vi "HFRR ADV v013 new software.vi"() -> ()   [LabVIEW 2025] (continued)
                              frame #4 {
                                n2582 = local write "Command"("HE;0" ("Command")) -> ()
                              }
                            }
                          }
                        }
                      }
                      frame True {
                      }
                    }
                    n2583 = local write "String 14"("Test will autostart once parameters reach the set value." ("String 14")) -> ()
                  }
                  frame True {
                    (unwired) FALSE ("Visible")
                    n2584 = property on="Stroke 2" class="DigNum (strict)"("Visible"=TRUE) -> ()  [unwired: 2 in, 2 out]
                    n2585 = property on="STOP 2" class="Bool (strict)"("Disabled"=u8 2) -> ()  [unwired: 2 in, 2 out]
                    n2586 = local write "String 14"(" Running....." ("String 14")) -> ()
                    n2587 = property on="Heater Button" class="Bool (strict)"("DisabledEnum"=T17."Disabled and Grayed Out" ("Disabled")) -> ()  [unwired: 2 in, 2 out]
                    n2588 = property on="Humidity" class="Bool (strict)"("DisabledEnum"=T17."Disabled and Grayed Out" ("Disabled")) -> ()  [unwired: 2 in, 2 out]
                    n2589 = case shown="True" "Start Time" {
                      selector: "Start Time" -> [_ w3108]
                      frame False {
                      }
                      frame True {
                        n2590 = Not(x=w3108) -> (.not. x?=w3107:bool)
                        n2591 = local write "Start Time"(w3107) -> ()
                        n2592 = local read "EVENT LOG"() -> (w3109:string)
                        n2593 = call "Event Log.vi"("Content"="Test in progress", "EVENT LOG"=w3109) -> ("EVENT LOG"=w3111:string)  [unwired: 8 in, 1 out]
                        n2594 = local write "EVENT LOG"(w3111) -> ()
                      }
                    }
                    n2595 = disable-structure shown="Enabled" {
                      disable-tunnel: [w3100 w3106] -> w3089
                      frame Disabled {
                        n2596 = local read "Set Hz"() -> (w3103:dbl)
                        n2597 = call <vilib>:"Uniform White Noise Waveform.vi"() -> ("signal out"=w3102:waveform(dbl))  [unwired: 10 in, 1 out]
                        n2598 = Random Number (0-1)() -> (number: 0 to 1=w3099:dbl)
                        n2599 = Add(x=w3103, y=w3102) -> (x+y=w3101:waveform(dbl))
                        n2600 = Multiply(x=ext 0.01 ("y"), y=w3099) -> (x*y=w3097:ext)
                        n2601 = Multiply(x=w3101, y=w3097) -> (x*y=w3100:waveform(ext))
                      }
                      frame Enabled {
                        n2602 = call-poly <vilib>:"Random Number (Range).vi"("lower bound (0)"=49.89, "upper bound (100)"=50.8) -> ("number"=w3106:dbl)  [unwired: 9 in]
                      }
                    }
                    "StartFlg" <- TRUE ("StartFlg")
                  }
                }
                n2603 = case shown="True" w3060 {
                  frame False {
                  }
                  frame True {
                    n2604 = local write "clk"(10.0 ("clk")) -> ()
                    n2605 = Get Date/Time In Seconds() -> (seconds since 1Jan1904=w3114:timestamp)
                    n2606 = To Double Precision Float(number=w3114) -> (double precision float=w3112:dbl)
                    n2607 = local write "acq timer"(w3112) -> ()
                    n2608 = local write "act save time"(w3112) -> ()
                  }
                }
                n2609 = call "Elapsed Time"("Time Target (s)"="Countdown", "Reset"=w3049) -> ("Elapsed Time (s)"=w3054:dbl, "Time has Elapsed"=w3052:bool)  [unwired: 10 in, 6 out]
                "Countdown 2" <- w3054
                n2610 = Subtract(x=w3054, y=2.0) -> (x-y=w3057:dbl)
                n2611 = Less?(x=w3057, y="Countdown") -> (x < y?=w3055:bool)
                n2612 = And(x=w3055, y=w3052) -> (x .and. y?=w3051:bool)
                n2613 = case shown="True" w3051 {
                  frame False {
                  }
                  frame True {
                    (unwired) dbl[] [] ("History Data")
                    n2614 = local write "Engage"(FALSE ("Engage")) -> ()
                    n2615 = local write "RUN"(TRUE ("RUN")) -> ()
                    n2616 = local read "Humidity ( %RH )"() -> (→"Rh Before":dbl)
                  }
                }
                n2617 = local read "Test \nStatus"() -> (w3047:bool)
                n2618 = Select(t=w3045, s=w3047, f=0.0) -> (s? t:f=w3046:dbl)
                n2619 = local write "Frequency ( Hz )"(w3046) -> ()
              }
              frame #1 {
                w3137 = 1000000.0 ("x")
                # "HC;1/0\nST;VALUE"
                # "Elapsed time\ncof\nstroke\nAir temp\nTemp\nHumidity"
                # "acq timer\n\nact save time"
                # "convert to microseconds"
                n2620 = local read "COUNT"() -> (w3120:i32)
                n2621 = local read "Rate"() -> (w3133:dbl)
                n2622 = Divide(x=w3137, y=w3133) -> (x/y=w3138:dbl)
                n2623 = Greater Or Equal?(x=w3120, y=250) -> (x >= y?=w3119:bool)
                n2624 = Get Date/Time In Seconds() -> (seconds since 1Jan1904=w3140:timestamp)
                n2625 = case shown="True" w3119 {
                  frame False {
                    n2626 = local read "COUNT"() -> (w3141:i32)
                    n2627 = Increment(x=w3141) -> (x+1=w3142:i32)
                    n2628 = local write "COUNT"(w3142) -> ()
                  }
                  frame True {
                    n2629 = local write "COUNT"(0 ("COUNT")) -> ()
                  }
                }
                n2630 = local read "Samplingtime 2"() -> (w3118:dbl)
                n2631 = local read "act save time"() -> (w3135:dbl)
                n2632 = Divide(x=w3138, y=w3137) -> (x/y=w3136:dbl)
                n2633 = To Double Precision Float(number=w3140) -> (double precision float=w3129:dbl)
                n2634 = Add(x=w3135, y=w3118) -> (x+y=w3134:dbl)
                n2635 = local read "acq timer"() -> (w3139:dbl)
                n2636 = local read "COUNT"() -> (w3122:i32)
                n2637 = Greater Or Equal?(x=w3129, y=w3134) -> (x >= y?=w3117:bool)
                n2638 = Multiply(x=w3136, y=w3122) -> (x*y=w3128:dbl)
                n2639 = Subtract(x=w3129, y=w3139) -> (x-y=w3131:dbl)
                n2640 = local read "Save"() -> (w3132:bool)
                n2641 = Add(x=w3131, y=w3128) -> (x+y=w3115:dbl)
                "Elapsed time 3" <- w3115
                n2642 = And(x=w3117, y=w3132) -> (x .and. y?=w3130:bool)
                n2643 = Divide(x=w3115, y=60.0) -> (x/y=w3126:dbl)
                n2644 = local read "Test \nStatus"() -> (w3116:bool)
                n2645 = local read "clk"() -> (w3123:dbl)
                n2646 = Equal?(x=w3123, y=10.0) -> (x = y?=w3125:bool)
                n2647 = case shown="True" w3130 {
                  tunnel: w3129 -> [_ w3253]
                  tunnel: [FALSE ("Boolean 2") TRUE ("Boolean 2")] -> _
                  frame False {
                  }
                  frame True {
                    w3207 = ";" ("Substring")
                    # "Pid out/\nFreq response value"
                    n2648 = local write "act save time"(w3253) -> ()
                    n2649 = local read "FILE"() -> (w3201:string)
                    n2650 = call "file check.vi"("file name in"=w3201) -> ("error out"=w3204:errorcluster, "file name out"=w3199:string)  [unwired: 9 in]
                    n2651 = local read "LVDT STROKE"() -> (w3196:dbl)
                    n2652 = local read "Add up Stroke"() -> (w3194:dbl)
                    n2653 = call "FILE PATH CREATION.vi"("error in"=w3204, "FILE NAME :"=w3199) -> ("FILE OUT"=w3202:path)  [unwired: 8 in, 1 out]
                    n2654 = Concatenate Strings(w3199, ".dgf" ("Substring")) -> (w3203:string)
                    n2655 = Subtract(x=w3196, y=w3194) -> (x-y=w3195:dbl)
                    n2656 = Absolute Value(x=w3195) -> (abs(x)=w3193:dbl)
                    n2657 = local read "FF 2"() -> (→"Frictional Force ( N )" →"Frictional Force ( N )":dbl)
                    n2658 = Build Path(base path=w3202, name or relative path=w3203) -> (appended path=w3198:path)
                    n2659 = local read "COF 2"() -> (w3212:dbl)
                    "cof" <- w3212
                    "Coefficient of Friction" <- w3212
                    "COF 4" <- w3212
                    "Coefficient of Friction" <- w3212
                    n2660 = local read "TEMP"() -> (w3215:dbl)
                    "Temp" <- w3215
                    "Temperature ( Deg C )" <- w3215
                    n2661 = local read "Humidity ( %RH )"() -> (w3214:dbl)
                    "Humidity ( %RH )" <- w3214
                    "Humidity ( %RH )" <- w3214
                    n2662 = local read "Frequency ( Hz )"() -> (w3221:dbl)
                    n2663 = call <vilib>:"Mean PtByPt.vi"("x"=w3193, "sample length"=10) -> ("mean"=w3192:dbl)  [unwired: 2 in, 1 out]
                    n2664 = local read "Elapsed time"() -> (w3246:dbl)
                    n2665 = local read "AIR TEMP"() -> (w3219:dbl)
                    n2666 = local read "PID-out"() -> (w3224:dbl)
                    n2667 = local write "Temperature ( Deg C )"(w3215) -> ()
                    n2668 = Number To Fractional String(number=w3192, width (-)=i16 9 ("precision (6)"), precision (6)=i16 6) -> (F-format string=w3239:string)  [unwired: 1 in]
                    n2669 = Number To Fractional String(number=w3219, width (-)=i16 9 ("precision (6)"), precision (6)=i16 3) -> (F-format string=w3238:string)  [unwired: 1 in]
                    n2670 = Number To Fractional String(number=w3215, width (-)=i16 9 ("precision (6)"), precision (6)=i16 3) -> (F-format string=w3235:string)  [unwired: 1 in]
                    n2671 = Number To Fractional String(number=w3214, width (-)=i16 9 ("precision (6)"), precision (6)=i16 3) -> (F-format string=w3232:string)  [unwired: 1 in]
                    n2672 = Number To Fractional String(number=0.0, width (-)=i16 9 ("precision (6)"), precision (6)=i16 3) -> (F-format string=w3229:string)  [unwired: 1 in]
                    n2673 = Number To Fractional String(number=w3224, width (-)=i16 9 ("precision (6)"), precision (6)=i16 3) -> (F-format string=w3225:string)  [unwired: 1 in]
                    n2674 = Number To Fractional String(number=w3221, width (-)=i16 9 ("precision (6)"), precision (6)=i16 3) -> (F-format string=w3220:string)  [unwired: 1 in]
                    n2675 = Number To Fractional String(number=w3212, width (-)=i16 9 ("precision (6)"), precision (6)=i16 6) -> (F-format string=w3247:string)  [unwired: 1 in]
                    n2676 = Number To Fractional String(number=w3246, width (-)=i16 14 ("precision (6)"), precision (6)=i16 3) -> (F-format string=w3248:string)  [unwired: 1 in]
                    n2677 = Bundle("y"=1.02, "mean"=w3192, "y"=0.98) -> (w3213:cluster{"y":dbl, "mean":dbl, "y":dbl})  [unwired: 1 in]
                    n2678 = Number To Fractional String(number="Ambient Humidity :", width (-)=i16 9 ("precision (6)"), precision (6)=i16 6) -> (F-format string=w3205:string)  [unwired: 1 in]
                    n2679 = local read "RUN"() -> (w3211:bool)
                    n2680 = case shown="True" w3211 {
                      tunnel: w3213 -> [_ w3258]
                      tunnel: w3192 -> [_ w3257]
                      tunnel: w3192 -> [_ w3255]
                      tunnel: w3192 -> [_ w3256]
                      frame False {
                      }
                      frame True {
                        "Stroke ( mm )" <- w3258
                        "Stroke ( mm )" <- w3258
                        "Stroke 4" <- w3257
                        "Stroke 3" <- w3255
                        "Stroke 2" <- w3256
                        "measured_stroke" <- w3255
                      }
                    }
                    n2681 = Concatenate Strings(w3248, w3207, w3247, w3207, w3239, w3207, w3238, w3207, w3235, w3207, w3232, w3207, w3229, w3207, w3225, w3207, w3220, w3207, w3205, "\r") -> (w3245:string)
                    n2682 = call <vilib>:"Write Characters To File.vi"("append to file? (new file:F)"=TRUE, "character string"=w3245, "file path (dialog if empty)"=w3198) -> ()  [unwired: 2 in, 1 out]
                    "refresh flag" <- TRUE ("refresh flag")
                  }
                }
                n2683 = case shown="True" w3116 {
                  tunnel: w3126 -> [_ w3152]
                  tunnel: w3131 -> [_ w3162]
                  tunnel: [0.0 w3158] -> _
                  tunnel: w3125 -> [_ w3157]
                  tunnel: [0.0 w3156] -> _
                  tunnel: w3115 -> [_ w3156]
                  tunnel: w3129 -> [w3145 _]
                  frame False {
                    n2684 = local write "acq timer"(w3145) -> ()
                    n2685 = local write "Test Duration Status"(0.0 ("Test Duration Status")) -> ()
                  }
                  frame True {
                    n2686 = local read "Set Hz"() -> (w3159:dbl)
                    n2687 = local write "Elapsed time"(w3152) -> ()
                    n2688 = local read "test time"() -> (w3151:dbl)
                    n2689 = Multiply(x=w3162, y=w3159) -> (x*y=w3161:dbl)
                    n2690 = case shown="False" w3157 {
                      tunnel: w3161 -> [w3163 _]
                      tunnel: [w3163 1.0] -> w3158
                      frame False {
                        n2691 = local write "Cycles elapsed"(w3163) -> ()
                      }
                      frame True {
                      }
                    }
                    n2692 = Greater?(x=w3152, y=w3151) -> (0:w3160:bool)
                    n2693 = Subtract(x=w3151, y=w3152) -> (x-y=w3150:dbl)
                    "time" <- w3150
                    n2694 = Multiply(x=w3150, y=60.0) -> (x*y=w3149:dbl)
                    n2695 = local write "Time Remaining"(w3149) -> ()
                    n2696 = local write "Remaining Time"(w3149) -> ()
                    n2697 = case shown="True" w3160 {
                      frame False {
                      }
                      frame True {
                        n2698 = stacked-sequence {
                          frame #0 {
                            w3168 = T17."Enabled" ("Disabled")
                            w3167 = FALSE ("TEST FILE NAM,E SAVED")
                            w3169 = "" ("FILE")
                            w3170 = TRUE ("Visible")
                            n2699 = local write "Humidity"(FALSE ("Humidity")) -> ()
                            n2700 = local write "RUN"(FALSE ("OK Button 2")) -> ()
                            n2701 = local write "Heater Button"(FALSE ("Heater Button")) -> ()
                            n2702 = local write "Auto Start Test"(FALSE ("Auto Start Test")) -> ()
                            n2703 = local write "TestCompFlg"(TRUE ("StpFlg")) -> ()
                            n2704 = local read "Humidity ( %RH )"() -> (→"Rh After":dbl)
                            n2705 = property on="STOP 2" class="Bool (strict)"("Disabled"=u8 0) -> ()  [unwired: 2 in, 2 out]
                            n2706 = local read "EVENT LOG"() -> (w3175:string)
                            n2707 = call "Event Log.vi"("Content"="Test Completed", "EVENT LOG"=w3175) -> ("EVENT LOG"=w3174:string)  [unwired: 8 in, 1 out]
                            n2708 = property on="RUN" class="Bool (strict)"("Visible"=w3170) -> ()  [unwired: 2 in, 2 out]
                            n2709 = property on="Auto Start Test" class="Bool (strict)"("Visible"=w3170) -> ()  [unwired: 2 in, 2 out]
                            n2710 = local write "Batch Ref Num :"(w3169) -> ()
                            n2711 = local write "FILE"(w3169) -> ()
                            n2712 = local write "EVENT LOG"(w3174) -> ()
                            n2713 = local write "TEST FILE NAM,E SAVED"(w3167) -> ()
                            n2714 = local write "Fuel Discription :"(w3169) -> ()
                            n2715 = local write "START TEMP"(w3167) -> ()
                            n2716 = local write "Remarks :"(w3169) -> ()
                            n2717 = local write "Main Dashboard Buttons"(T1."Imaging" ("Main Dashboard Buttons")) -> ()
                            n2718 = local write "Main Tab"(T2."Adv Scar" ("Main Tab")) -> ()
                            n2719 = property on="FRICVALZ 2" class="Bool (strict)"("DisabledEnum"=w3168) -> ()  [unwired: 2 in, 2 out]
                            n2720 = property on="FRICVALZ 3" class="Bool (strict)"("DisabledEnum"=w3168) -> ()  [unwired: 2 in, 2 out]
                            n2721 = property on="FRICVALZ 4" class="Bool (strict)"("DisabledEnum"=w3168) -> ()  [unwired: 2 in, 2 out]
                          }
                          frame #1 {
                            n2722 = Wait (ms)(milliseconds to wait=u32 1500) -> ()  [unwired: 1 out]
                          }
                          frame #2 {
                            n2723 = local write "Command"("VC;0") -> ()
                          }
                          frame #3 {
                            n2724 = Wait (ms)(milliseconds to wait=u32 1500) -> ()  [unwired: 1 out]
                          }
                          frame #4 {
                            n2725 = local write "Command"("VC;0") -> ()
                          }
                          frame #5 {
                            n2726 = Wait (ms)(milliseconds to wait=u32 1500) -> ()  [unwired: 1 out]
                          }
                          frame #6 {
                            n2727 = local write "Command"("ST;0") -> ()
                          }
                          frame #7 {
                            n2728 = local write "measured_stroke"(0.0 ("measured_stroke")) -> ()
                            n2729 = Wait (ms)(milliseconds to wait=u32 1500) -> ()  [unwired: 1 out]
                          }
                          frame #8 {
                            n2730 = local write "Command"("HE;0") -> ()
                          }
                        }
                      }
                    }
                    n2731 = Divide(x=w3152, y=w3151) -> (x/y=w3155:dbl)
                    n2732 = Multiply(x=w3155, y=100.0) -> (x*y=w3153:dbl)
                    n2733 = local write "Test Duration Status"(w3153) -> ()
                  }
                }
              }
              frame #2 {
                n2734 = case shown="True" "Heater Button" {
                  tunnel: [0.0 ("output") w3281] -> w3259
                  frame False {
                    w3262 = TRUE ("tmpchk")
                    n2735 = local read "TEMP"() -> (w3263:dbl)
                    n2736 = local write "Temp ini"(w3263) -> ()
                    n2737 = local write "Reset 4"(w3262) -> ()
                    n2738 = local write "tmpchk"(w3262) -> ()
                    n2739 = local write "reinit"(TRUE ("reinit")) -> ()
                    n2740 = local write "manual temp log"(TRUE ("manual temp log")) -> ()
                  }
                  frame True {
                    # "Logic to turn off\nthe heater when \ntemp is not rising.\nTime - 60 sec\nDelta t- 5°c"
                    n2741 = local read "Temp ini"() -> (w3270:dbl)
                    n2742 = local read "Auto Start Test"() -> (w3266:bool)
                    n2743 = Less?(x=w3270, y=53.0) -> (x < y?=w3268:bool)
                    n2744 = case shown="False" w3266 {
                      frame False {
                        n2745 = local read "Set Temp"() -> (w3290:dbl)
                        n2746 = local read "TEMP"() -> (w3289:dbl)
                        n2747 = Subtract(x=w3290, y=w3289) -> (x-y=w3288:dbl)
                        n2748 = Absolute Value(x=w3288) -> (abs(x)=w3287:dbl)
                        n2749 = Less?(x=w3287, y=0.5) -> (x < y?=w3285:bool)
                        n2750 = case shown="True" w3285 {
                          tunnel: "manual temp log" -> [_ w3291]
                          frame False {
                          }
                          frame True {
                            n2751 = case shown="True" w3291 {
                              selector: w3291 -> [_ w3292]
                              frame False {
                              }
                              frame True {
                                # "#Event log"
                                n2752 = Not(x=w3292) -> (.not. x?=w3293:bool)
                                n2753 = local write "manual temp log"(w3293) -> ()
                                n2754 = local read "EVENT LOG"() -> (w3296:string)
                                n2755 = call "Event Log.vi"("Content"="Target Temperature reached", "EVENT LOG"=w3296) -> ("EVENT LOG"=w3295:string)  [unwired: 8 in, 1 out]
                                n2756 = local write "EVENT LOG"(w3295) -> ()
                              }
                            }
                          }
                        }
                      }
                      frame True {
                        n2757 = local write "manual temp log"(TRUE ("manual temp log")) -> ()
                      }
                    }
                    n2758 = And(x="tmpchk", y=w3268) -> (x .and. y?=w3271:bool)
                    n2759 = case shown="True" w3271 {
                      frame False {
                      }
                      frame True {
                        n2760 = call "Elapsed Time8"("Time Target (s)"=300.0, "Reset"="Reset 4") -> ("Time has Elapsed"=w3298:bool)  [unwired: 10 in, 7 out]
                        n2761 = flat-sequence {
                          tunnel: w3298 -> [_]
                          frame #0 {
                            n2762 = local write "Reset 4"(FALSE ("Reset 4")) -> ()
                          }
                        }
                        n2763 = case shown="True" w3298 {
                          frame False {
                          }
                          frame True {
                            n2764 = local read "Temp ini"() -> (w3305:dbl)
                            n2765 = Add(x=w3305, y=5.0) -> (x+y=w3303:dbl)
                            n2766 = local read "TEMP"() -> (w3306:dbl)
                            n2767 = Greater?(x=w3306, y=w3303) -> (0:w3304:bool)
                            n2768 = case shown="False" w3304 {
                              frame False {
                                n2769 = local write "Heater Button"(FALSE ("Heater Button")) -> ()
                              }
                              frame True {
                                n2770 = local write "tmpchk"(FALSE ("tmpchk")) -> ()
                              }
                            }
                          }
                        }
                      }
                    }
                    n2771 = local read "Set Temp"() -> (w3279:dbl)
                    n2772 = local read "TEMP"() -> (w3273:dbl)
                    n2773 = call-poly <vilib>:"PID.vi"("reinitialize? (F)"="reinit", "dt (s)"=-1.0, "process variable"=w3273, "setpoint"=w3279) -> ("output"=w3276:dbl)  [unwired: 6 in, 1 out]
                    n2774 = Subtract(x=w3279, y=w3273) -> (x-y=w3280:dbl)
                    n2775 = Add(x=w3279, y=0.5) -> (x+y=w3277:dbl)
                    n2776 = Greater Or Equal?(x=w3273, y=w3277) -> ()  [unwired: 1 out]
                    n2777 = Select(t=0.0, s=FALSE, f=w3276) -> (s? t:f=w3275:dbl)
                    "PID output" <- w3275
                    n2778 = flat-sequence {
                      tunnel: w3275 -> [w3309]
                      tunnel: [w3309] -> w3281
                      frame #0 {
                        n2779 = local write "reinit"(FALSE ("reinit")) -> ()
                      }
                    }
                    n2780 = Bundle(w3280, "output"=w3275, "TEMP"=w3273) -> ()  [unwired: 1 in, 1 out]
                  }
                }
                "PID-out" <- w3259
              }
              frame #3 {
                n2781 = local read "TEMP"() -> (w3311:dbl)
                n2782 = Greater Or Equal?(x=w3311, y="Set Temp 2") -> (x >= y?=w3316:bool)
                n2783 = case shown="True" w3316 {
                  tunnel: [FALSE TRUE] -> w3314
                  frame False {
                  }
                  frame True {
                  }
                }
                "Status 13" <- w3314
                n2784 = And(x=w3314, y="trip1 8") -> (x .and. y?=w3313:bool)
                n2785 = case shown="True" w3313 {
                  frame False {
                    n2786 = local write "Heater Trip Temp"(TRUE ("Heater Trip Temp")) -> ()
                  }
                  frame True {
                    w3319 = FALSE ("OK Button 2")
                    n2787 = case shown="True" "Heater Trip Temp" {
                      selector: "Heater Trip Temp" -> [_ w3321]
                      frame False {
                      }
                      frame True {
                        n2788 = Not(x=w3321) -> (.not. x?=w3320:bool)
                        n2789 = local read "EVENT LOG"() -> (w3324:string)
                        n2790 = local write "Heater Trip Temp"(w3320) -> ()
                        n2791 = call "Event Log.vi"("Content"="Heater Trip", "EVENT LOG"=w3324) -> ("EVENT LOG"=w3323:string)  [unwired: 8 in, 1 out]
                        n2792 = local write "EVENT LOG"(w3323) -> ()
                      }
                    }
                    n2793 = local write "RUN"(w3319) -> ()
                    n2794 = property on="Auto Start Test" class="Bool (strict)"("Value"=w3319) -> ()  [unwired: 2 in, 2 out]
                    n2795 = local write "Heater Button"(w3319) -> ()
                  }
                }
              }
            }
            n2796 = case shown="False" w3040 {
              frame False {
                n2797 = disable-structure shown="Disabled" {
                  frame Disabled {
                    n2798 = stacked-sequence {
                      frame #0 {
                        n2799 = local write "RUN"(FALSE ("OK Button 2")) -> ()
                      }
                      frame #1 {
                      }
                    }
                  }
                  frame Enabled {
                  }
                }
              }
              frame True {
              }
            }
          }
        }
        n2800 = local read "airtempflg"() -> (w2832:bool)
        n2801 = Or(x=w2832, y=w2830) -> (x .or. y?=w2833:bool)
        n2802 = Insert Into Array(array=string[] ["Air Temperature has reached set value,", "Humidity has reached set value,", "Sample Temperaturehas reached set value,", ""], index=0, new element="") -> (w2818:string[])
        n2803 = Build Array(w2823, w2822, w2821) -> (w2819:i32[])
        n2804 = disable-structure shown="Disabled" {
          disable-tunnel: w2833 -> [w2910 _]
          disable-tunnel: w2828 -> [w2909 _]
          disable-tunnel: w2826 -> [w2908 _]
          frame Disabled {
            n2805 = Compound Arithmetic op=AND(w2910, w2909, w2908) -> ()  [unwired: 1 out]
            n2806 = case shown="True" {
              selector: _ -> [_ _]
              frame False {
              }
              frame True {
                w2911 = FALSE ("autostrtflg")
                n2807 = local write "RUN"(TRUE ("RUN")) -> ()
                n2808 = local write "autostrtflg"(w2911) -> ()
                n2809 = local write "autostart"(w2911) -> ()
                n2810 = local write "String 14"(" Running....." ("String 14")) -> ()
              }
            }
          }
          frame Enabled {
          }
        }
        n2811 = for {
          tunnel: w2819 -> [w2961] mode=indexing
          tunnel: w2818 -> [w2960]
          shift-right: [w2957] -> w2817
          shift-left: "" -> [w2959]
          n2812 = Index Array(array=w2960, index=w2961) -> (element=w2958:string)
          n2813 = Concatenate Strings(w2958, w2959) -> (w2957:string)
        }
        n2814 = local write "autostart 2"(w2817) -> ()
        n2815 = local read "Reset Graph"() -> (w2806:bool)
        n2816 = case shown="True" w2806 {
          selector: w2806 -> [_ w2860]
          frame False {
          }
          frame True {
            w2874 = 0.0 ("X Scale.Range:Maximum")
            n2817 = Not(x=w2860) -> (.not. x?=w2859:bool)
            n2818 = local write "Reset Graph"(w2859) -> ()
            n2819 = property on="Electrical Contact Resistance ( % )" class="WFChart (strict)"("XScale.Maximum"=600.0 ("X Scale.Range:Maximum"), "XScale.Minimum"=0.0 ("X Scale.Range:Minimum"), "YScale.Maximum"=100.0 ("Y Scale.Range:Maximum"), "YScale.Minimum"=0.0 ("Y Scale.Range:Minimum")) -> ()  [unwired: 2 in, 2 out]
            n2820 = property on="Frictional Force ( N )" class="WFChart (strict)"("XScale.Maximum"=600.0 ("X Scale.Range:Maximum"), "XScale.Minimum"=0.0 ("X Scale.Range:Minimum"), "YScale.Maximum"=100.0 ("Y Scale.Range:Maximum"), "YScale.Minimum"=0.0 ("Y Scale.Range:Minimum")) -> ()  [unwired: 2 in, 2 out]
            n2821 = property on="Temperature ( Deg C )" class="WFChart (strict)"("XScale.Maximum"=600.0 ("X Scale.Range:Maximum"), "XScale.Minimum"=0.0 ("X Scale.Range:Minimum"), "YScale.Maximum"=100.0 ("Y Scale.Range:Maximum"), "YScale.Minimum"=0.0 ("Y Scale.Range:Minimum")) -> ()  [unwired: 2 in, 2 out]
            n2822 = property on="Humidity ( %RH )" class="WFChart (strict)"("XScale.Maximum"=600.0 ("X Scale.Range:Maximum"), "XScale.Minimum"=0.0 ("X Scale.Range:Minimum"), "YScale.Maximum"=100.0 ("Y Scale.Range:Maximum"), "YScale.Minimum"=0.0 ("Y Scale.Range:Minimum")) -> ()  [unwired: 2 in, 2 out]
            n2823 = property on="Stroke ( mm )" class="WFChart (strict)"("XScale.Maximum"=600.0 ("X Scale.Range:Maximum"), "XScale.Minimum"=0.0 ("X Scale.Range:Minimum"), "YScale.Maximum"=100.0 ("Y Scale.Range:Maximum"), "YScale.Minimum"=0.0 ("Y Scale.Range:Minimum")) -> ()  [unwired: 2 in, 2 out]
            n2824 = property on="Coefficient of Friction" class="WFChart (strict)"("XScale.Maximum"=600.0 ("X Scale.Range:Maximum"), "XScale.Minimum"=0.0 ("X Scale.Range:Minimum"), "YScale.Maximum"=100.0 ("Y Scale.Range:Maximum"), "YScale.Minimum"=0.0 ("Y Scale.Range:Minimum")) -> ()  [unwired: 2 in, 2 out]
            n2825 = property on="Electrical Contact Resistance ( % )" class="WFChart (strict)"("XScale.Minimum"=0.0 ("X Scale.Range:Minimum"), "XScale.Maximum"=600.0 ("X Scale.Range:Maximum"), "YScale.Minimum"=0.0 ("Y Scale.Range:Minimum"), "YScale.Maximum"=100.0 ("Y Scale.Range:Maximum")) -> ()  [unwired: 2 in, 2 out]
            n2826 = property on="Temperature ( Deg C )" class="WFChart (strict)"("XScale.Minimum"=0.0 ("X Scale.Range:Minimum"), "XScale.Maximum"=600.0 ("X Scale.Range:Maximum"), "YScale.Minimum"=0.0 ("Y Scale.Range:Minimum"), "YScale.Maximum"=100.0 ("Y Scale.Range:Maximum")) -> ()  [unwired: 2 in, 2 out]
            n2827 = property on="Coefficient of Friction" class="WFChart (strict)"("XScale.Minimum"=0.0 ("X Scale.Range:Minimum"), "XScale.Maximum"=600.0 ("X Scale.Range:Maximum"), "YScale.Maximum"=1.0 ("X Scale.Range:Minimum"), "YScale.Minimum"=0.0 ("X Scale.Range:Minimum")) -> ()  [unwired: 2 in, 2 out]
            n2828 = property on="Frictional Force ( N )" class="WFChart (strict)"("XScale.Maximum"=600.0 ("X Scale.Range:Maximum"), "XScale.Minimum"=w2874, "YScale.Maximum"=10.0 ("Y Scale.Range:Maximum"), "YScale.Minimum"=w2874) -> ()  [unwired: 2 in, 2 out]
            n2829 = property on="Stroke ( mm )" class="WFChart (strict)"("XScale.Maximum"=600.0 ("X Scale.Range:Maximum"), "XScale.Minimum"=0.0 ("X Scale.Range:Minimum"), "YScale.Maximum"=100.0 ("Y Scale.Range:Maximum"), "YScale.Minimum"=0.0 ("Y Scale.Range:Minimum")) -> ()  [unwired: 2 in, 2 out]
            n2830 = property on="Humidity ( %RH )" class="WFChart (strict)"("XScale.Maximum"=600.0 ("X Scale.Range:Maximum"), "XScale.Minimum"=0.0 ("X Scale.Range:Minimum"), "YScale.Maximum"=100.0 ("Y Scale.Range:Maximum"), "YScale.Minimum"=0.0 ("Y Scale.Range:Minimum")) -> ()  [unwired: 2 in, 2 out]
          }
        }
      }
      frame "Compare Files" {
        # "Elapsed time\ncof\nstroke\nAir temp\nTemp\nHumidity"
        n2831 = case shown="True" "RSTV1 2" {
          frame False {
          }
          frame True {
            n2832 = property on="Humidity ( %RH )" class="XYGraph (strict)"("Y Scale.Display Format:Precision"=u8 0 ("Y Scale.Format & Precision:Precision")) -> ()  [unwired: 2 in, 2 out]
            n2833 = property on="Humidity ( %RH )" class="XYGraph (strict)"("X Scale.Range:Minimum"=0.0, "X Scale.Range:Maximum"=75.0, "Y Scale.Range:Minimum"=48.0, "Y Scale.Range:Maximum"=58.0) -> ()  [unwired: 2 in, 2 out]
          }
        }
        n2834 = case shown="True" "RST CP 2" {
          frame False {
          }
          frame True {
            n2835 = property on="XY Graph 13" class="XYGraph (strict)"("Y Scale.Display Format:Precision"=u8 0 ("Y Scale.Format & Precision:Precision")) -> ()  [unwired: 2 in, 2 out]
            n2836 = property on="XY Graph 13" class="XYGraph (strict)"("X Scale.Range:Minimum"=0.0, "X Scale.Range:Maximum"=75.0, "Y Scale.Range:Minimum"=0.0, "Y Scale.Range:Maximum"=100.0) -> ()  [unwired: 2 in, 2 out]
          }
        }
        n2837 = case shown="True" "RST CP" {
          frame False {
          }
          frame True {
            n2838 = property on="Sample Temperature ( °C )" class="XYGraph (strict)"("Y Scale.Display Format:Precision"=u8 2 ("Y Scale.Format & Precision:Precision")) -> ()  [unwired: 2 in, 2 out]
            n2839 = property on="Sample Temperature ( °C )" class="XYGraph (strict)"("X Scale.Range:Minimum"=0.0, "X Scale.Range:Maximum"=75.0, "Y Scale.Range:Minimum"=58.0, "Y Scale.Range:Maximum"=62.0) -> ()  [unwired: 2 in, 2 out]
          }
        }
        n2840 = case shown="True" "RSTV1 3" {
          frame False {
          }
          frame True {
            n2841 = property on="Air Temperature  ( °C )" class="XYGraph (strict)"("Y Scale.Display Format:Precision"=u8 2 ("Y Scale.Format & Precision:Precision")) -> ()  [unwired: 2 in, 2 out]
            n2842 = property on="Air Temperature  ( °C )" class="XYGraph (strict)"("X Scale.Range:Minimum"=0.0 ("Y Scale.Range:Minimum"), "X Scale.Range:Maximum"=75.0 ("Y Scale.Range:Maximum"), "Y Scale.Range:Minimum"=20.0 ("X Scale.Range:Minimum"), "Y Scale.Range:Maximum"=26.0 ("X Scale.Range:Maximum")) -> ()  [unwired: 2 in, 2 out]
          }
        }
        n2843 = case shown="True" "RSTV1 4" {
          frame False {
          }
          frame True {
            n2844 = property on="Stroke ( mm )" class="XYGraph (strict)"("Y Scale.Display Format:Precision"=u8 2 ("Y Scale.Format & Precision:Precision")) -> ()  [unwired: 2 in, 2 out]
            n2845 = property on="Stroke ( mm )" class="XYGraph (strict)"("X Scale.Range:Minimum"=0.0 ("Y Scale.Range:Maximum"), "X Scale.Range:Maximum"=75.0 ("X Scale.Range:Minimum"), "Y Scale.Range:Minimum"=0.98, "Y Scale.Range:Maximum"=1.02) -> ()  [unwired: 2 in, 2 out]
          }
        }
        n2846 = case shown="True" "rstv2" {
          frame False {
          }
          frame True {
            n2847 = property on="Coefficient Of Friction" class="XYGraph (strict)"("Y Scale.Display Format:Precision"=u8 3 ("Y Scale.Format & Precision:Precision")) -> ()  [unwired: 2 in, 2 out]
            n2848 = property on="Coefficient Of Friction" class="XYGraph (strict)"("X Scale.Range:Minimum"=0.0 ("Y Scale.Range:Maximum"), "X Scale.Range:Maximum"=75.0, "Y Scale.Range:Minimum"=0.0, "Y Scale.Range:Maximum"=1.0 ("X Scale.Range:Minimum")) -> ()  [unwired: 2 in, 2 out]
          }
        }
        n2849 = case shown="True" "RST CP 3" {
          frame False {
          }
          frame True {
            n2850 = property on="Air Temp ( °C ) vs Humidity ( % RH )" class="XYGraph (strict)"("X Scale.Range:Minimum"=18.0, "X Scale.Range:Maximum"=28.0 ("X Scale.Range:Minimum"), "Y Scale.Range:Minimum"=30.0 ("X Scale.Range:Minimum"), "Y Scale.Range:Maximum"=70.0 ("X Scale.Range:Minimum")) -> ()  [unwired: 2 in, 2 out]
          }
        }
        n2851 = case shown="True" "OPEN 1" {
          frame False {
          }
          frame True {
            (unwired) 0  # existing file
            w3600 = "Choose a datalog file to open"  # prompt
            n2852 = local write "OPEN 1"(FALSE ("OPEN 1")) -> ()
            n2853 = String To Path(string="C:\\LAB-IQ\\Data\\") -> (path=w3585:path)
            n2854 = File Dialog(6:"*.dgf" ("pattern"), 7:w3600, 11:w3585) -> (0:w3583:errorcluster, 3:w3591:path)  [unwired: 4 in, 2 out]
            n2855 = Unbundle(w3583) -> ()  [unwired: 3 out]
            n2856 = Strip Path(path=w3591) -> (name=w3590:string)  [unwired: 1 out]
            n2857 = Path To String(path=w3591) -> (string=w3586:string)
            "string1" <- w3586
            n2858 = Match Pattern(string=w3590, regular expression=".dgf") -> (before substring=→"String Control":string)  [unwired: 1 in, 3 out]
            n2859 = Match Pattern(string=w3586, regular expression=".dgf" ("substring (\"\")")) -> (before substring=w3596:string)  [unwired: 1 in, 3 out]
            n2860 = Concatenate Strings(w3596, ".duf" ("Substring")) -> (w3592:string)
            n2861 = String To Path(string=w3592) -> (path=w3597:path)
            n2862 = call <vilib>:"Read Characters From File.vi"("file path (dialog if empty)"=w3597, "start of read offset (chars.:0)"=60 ("start of read offset (chars.: 0)")) -> ("character string"=→"String Control 2":string)  [unwired: 4 in, 3 out]
          }
        }
        n2863 = case shown="True" "OPEN 2" {
          frame False {
          }
          frame True {
            (unwired) 0  # existing file
            w3618 = "Choose a datalog file to open"  # prompt
            n2864 = local write "OPEN 2"(FALSE ("OPEN 1")) -> ()
            n2865 = String To Path(string="C:\\LAB-IQ\\Data\\") -> (path=w3603:path)
            n2866 = File Dialog(6:"*.dgf" ("pattern"), 7:w3618, 11:w3603) -> (0:w3601:errorcluster, 3:w3609:path)  [unwired: 4 in, 2 out]
            n2867 = Unbundle(w3601) -> ()  [unwired: 3 out]
            n2868 = Strip Path(path=w3609) -> (name=w3607:string)  [unwired: 1 out]
            n2869 = Path To String(path=w3609) -> (string=w3604:string)
            "string1 2" <- w3604
            n2870 = Match Pattern(string=w3607, regular expression=".dgf") -> (before substring=→"String Control 3":string)  [unwired: 1 in, 3 out]
            n2871 = Match Pattern(string=w3604, regular expression=".dgf" ("substring (\"\")")) -> (before substring=w3615:string)  [unwired: 1 in, 3 out]
            n2872 = Concatenate Strings(w3615, ".duf" ("Substring")) -> (w3612:string)
            n2873 = String To Path(string=w3612) -> (path=w3610:path)
            n2874 = call <vilib>:"Read Characters From File.vi"("file path (dialog if empty)"=w3610, "start of read offset (chars.:0)"=60 ("start of read offset (chars.: 0)")) -> ("character string"=→"String Control 4":string)  [unwired: 4 in, 3 out]
          }
        }
        n2875 = case shown="True" "OPEN 3" {
          frame False {
          }
          frame True {
            (unwired) 0  # existing file
            w3636 = "Choose a datalog file to open"  # prompt
            n2876 = local write "OPEN 3"(FALSE ("OPEN 1")) -> ()
            n2877 = String To Path(string="C:\\LAB-IQ\\Data\\") -> (path=w3621:path)
            n2878 = File Dialog(6:"*.dgf" ("pattern"), 7:w3636, 11:w3621) -> (0:w3619:errorcluster, 3:w3627:path)  [unwired: 4 in, 2 out]
            n2879 = Unbundle(w3619) -> ()  [unwired: 3 out]
            n2880 = Strip Path(path=w3627) -> (name=w3625:string)  [unwired: 1 out]
            n2881 = Path To String(path=w3627) -> (string=w3622:string)
            "string1 3" <- w3622
            n2882 = Match Pattern(string=w3625, regular expression=".dgf") -> (before substring=→"String Control 5":string)  [unwired: 1 in, 3 out]
            n2883 = Match Pattern(string=w3622, regular expression=".dgf" ("substring (\"\")")) -> (before substring=w3632:string)  [unwired: 1 in, 3 out]
            n2884 = Concatenate Strings(w3632, ".duf" ("Substring")) -> (w3629:string)
            n2885 = String To Path(string=w3629) -> (path=w3633:path)
            n2886 = call <vilib>:"Read Characters From File.vi"("file path (dialog if empty)"=w3633, "start of read offset (chars.:0)"=60 ("start of read offset (chars.: 0)")) -> ("character string"=→"String Control 6":string)  [unwired: 4 in, 3 out]
          }
        }
        n2887 = case shown="True" "OPEN 4" {
          frame False {
          }
          frame True {
            (unwired) 0  # existing file
            w3654 = "Choose a datalog file to open"  # prompt
            n2888 = local write "OPEN 4"(FALSE ("OPEN 1")) -> ()
            n2889 = String To Path(string="C:\\LAB-IQ\\Data\\") -> (path=w3639:path)
            n2890 = File Dialog(6:"*.dgf" ("pattern"), 7:w3654, 11:w3639) -> (0:w3637:errorcluster, 3:w3645:path)  [unwired: 4 in, 2 out]
            n2891 = Unbundle(w3637) -> ()  [unwired: 3 out]
            n2892 = Strip Path(path=w3645) -> (name=w3643:string)  [unwired: 1 out]
            n2893 = Path To String(path=w3645) -> (string=w3640:string)
            "string1 4" <- w3640
            n2894 = Match Pattern(string=w3643, regular expression=".dgf") -> (before substring=→"String Control 7":string)  [unwired: 1 in, 3 out]
            n2895 = Match Pattern(string=w3640, regular expression=".dgf" ("substring (\"\")")) -> (before substring=w3650:string)  [unwired: 1 in, 3 out]
            n2896 = Concatenate Strings(w3650, ".duf" ("Substring")) -> (w3647:string)
            n2897 = String To Path(string=w3647) -> (path=w3651:path)
            n2898 = call <vilib>:"Read Characters From File.vi"("file path (dialog if empty)"=w3651, "start of read offset (chars.:0)"=60 ("start of read offset (chars.: 0)")) -> ("character string"=→"String Control 8":string)  [unwired: 4 in, 3 out]
          }
        }
      }
      frame "About" {
        # "Elapsed time\ncof\nstroke\nmean pos\nTemp\nHumidity"
        n2899 = disable-structure shown="Disabled" {
          frame Disabled {
            n2900 = case shown="True" "Export" {
              frame False {
              }
              frame True {
                w3676 = "                                      " ("string")
                w3678 = "\r"
                (unwired) i16 6 ("width (-)")
                w3755 = "\r"
                w3687 = "\r"
                n2901 = local write "Export"(FALSE ("Export")) -> ()
                n2902 = local read "String 29"() -> (w3724:string)
                n2903 = local read "String 34"() -> (w3712:string)
                n2904 = local read "String 35"() -> (w3707:string)
                n2905 = local read "String 37"() -> (w3703:string)
                n2906 = local read "String 36"() -> (w3700:string)
                n2907 = local read "String 38"() -> (w3697:string)
                n2908 = local read "String 39"() -> (w3694:string)
                n2909 = Match Pattern(string=w3724, regular expression=".dwm") -> (before substring=w3720:string)  [unwired: 1 in, 3 out]
                "before substring" <- w3720
                n2910 = local read "S 38"() -> (w3715:string)
                n2911 = local read "S 39"() -> (w3708:string)
                n2912 = local read "Temperature before test 2"() -> (w3744:dbl)
                n2913 = local read "Temperature after test 2"() -> (w3749:dbl)
                n2914 = local read "Humidity before test 2"() -> (w3730:dbl)
                n2915 = local read "Humidity after test 2"() -> (w3745:dbl)
                n2916 = local read "MWSD 2"() -> (w3741:dbl)
                n2917 = local read "WS1.4 2"() -> (w3757:dbl)
                n2918 = local read "HCF 2"() -> (w3753:dbl)
                n2919 = local read "AVP 2"() -> (w3742:dbl)
                n2920 = Concatenate Strings("1," ("string"), w3715) -> (w3714:string)
                n2921 = Concatenate Strings("2," ("string"), w3712) -> (w3711:string)
                n2922 = Concatenate Strings("3," ("string"), w3708) -> (w3710:string)
                n2923 = Concatenate Strings("4," ("string"), w3707) -> (w3706:string)
                n2924 = Concatenate Strings("5," ("string"), w3703) -> (w3704:string)
                n2925 = Concatenate Strings("6," ("string"), w3700) -> (w3701:string)
                n2926 = Concatenate Strings("7," ("string"), w3697) -> (w3698:string)
                n2927 = Concatenate Strings("8," ("string"), w3694) -> (w3695:string)
                n2928 = local read "Sample ID"() -> (w3762:string)
                n2929 = case shown="\"xlx\"" "Select File Type" {
                  tunnel: w3720 -> [w3765 w3767 w3769]
                  tunnel: [w3763 w3768 w3770] -> w3719
                  frame "xlx" {
                    n2930 = Concatenate Strings(w3765, ".xls" ("string")) -> (w3763:string)
                  }
                  frame "csv" {
                    n2931 = Concatenate Strings(w3767, ".csv" ("string")) -> (w3768:string)
                  }
                  frame "txt" {
                    n2932 = Concatenate Strings(w3769, ".txt" ("string")) -> (w3770:string)
                  }
                }
                n2933 = local read "Test Date"() -> (w3761:string)
                n2934 = local read "String 45"() -> (w3675:string)
                n2935 = local read "String 31"() -> (w3760:string)
                n2936 = local read "String 32"() -> (w3759:string)
                n2937 = local read "TITTLE"() -> (w3683:string)
                n2938 = Number To Fractional String(number=w3730, width (-)=i16 6, precision (6)=i16 2) -> (F-format string=w3729:string)  [unwired: 1 in]
                n2939 = Number To Fractional String(number=w3744, width (-)=i16 6, precision (6)=i16 2) -> (F-format string=w3750:string)  [unwired: 1 in]
                n2940 = Number To Fractional String(number=w3745, width (-)=i16 6, precision (6)=i16 2) -> (F-format string=w3743:string)  [unwired: 1 in]
                n2941 = Number To Fractional String(number=w3749, width (-)=i16 6, precision (6)=i16 2) -> (F-format string=w3748:string)  [unwired: 1 in]
                n2942 = Number To Fractional String(number=w3741, width (-)=i16 6, precision (6)=i16 2) -> (F-format string=w3739:string)  [unwired: 1 in]
                n2943 = Number To Fractional String(number=w3742, width (-)=i16 6, precision (6)=i16 2) -> (F-format string=w3740:string)  [unwired: 1 in]
                n2944 = Number To Fractional String(number=w3753, width (-)=i16 6, precision (6)=i16 2) -> (F-format string=w3754:string)  [unwired: 1 in]
                n2945 = Number To Fractional String(number=w3757, precision (6)=i16 2) -> (F-format string=w3758:string)  [unwired: 2 in]
                n2946 = local read "s.NO"() -> (w3677:string)
                n2947 = Concatenate Strings("=" ("string"), w3683) -> (w3682:string)
                n2948 = Concatenate Strings("S.No," ("string"), "                                       Parameters" ("string")) -> (w3688:string)
                n2949 = Concatenate Strings(w3755, w3714, w3729, w3755, w3711, w3750, w3755, w3710, w3743, w3755, w3706, w3748, w3755, w3704, w3739, w3755, w3701, w3740, w3755, w3698, w3754, w3755, w3695, w3758) -> (w3717:string)
                n2950 = Concatenate Strings(w3687, "," ("string"), w3675, w3677, w3676, w3759, w3762, w3676, w3760, w3761, w3687) -> (w3685:string)
                n2951 = local read "Tested by"() -> (w3691:string)
                n2952 = local read "String 33"() -> (w3692:string)
                n2953 = Concatenate Strings("," ("string"), "                                                                             " ("string")) -> (w3680:string)
                n2954 = Concatenate Strings(w3682, w3678, w3685, w3678, w3688, w3717, w3678, w3680, w3692, w3691) -> (→"export":string)
                n2955 = String To Path(string=w3719) -> (path=w3726:path)
                n2956 = local read "export"() -> (w3721:string)
                n2957 = call <vilib>:"Write Characters To File.vi"("append to file? (new file:F)"=FALSE, "character string"=w3721, "file path (dialog if empty)"=w3726) -> ()  [unwired: 2 in, 1 out]
              }
            }
          }
          frame Enabled {
          }
        }
        n2958 = case shown="True" "OK Button 17" {
          frame False {
          }
          frame True {
            (unwired) 0  # existing file
            w3979 = "Choose a datalog file to open"  # prompt
            n2959 = local write "OK Button 17"(FALSE ("OK Button 17")) -> ()
            n2960 = local read "String"() -> (w3974:string)
            n2961 = String To Path(string=w3974) -> (path=w3975:path)
            n2962 = File Dialog(6:"*.duf" ("pattern"), 7:w3979, 11:w3975) -> (0:w3966:errorcluster, 3:w3985:path)  [unwired: 4 in, 2 out]
            n2963 = Unbundle(w3966) -> ()  [unwired: 3 out]
            n2964 = Open/Create/Replace File "Open File"(file path (use dialog)=w3985) -> (refnum out=w3977:refnum<file>)  [unwired: 5 in, 2 out]
            n2965 = Strip Path(path=w3985) -> (name=w3983:string)  [unwired: 1 out]
            n2966 = Path To String(path=w3985) -> (string=w3968:string)
            n2967 = while {
              tunnel: w3977 -> [w3989]
              i -> [w3986]
              stop <- w3987 continue-if-true
              (unwired) TRUE ("line mode (F)")
              n2968 = Read from Text File "Read File"(file (use dialog)=w3989) -> (text=w3988:string)  [unwired: 3 in, 3 out]
              n2969 = local write "Numeric 16"(w3986) -> ()
              n2970 = String Length(string=w3988) -> (length=w3991:i32)
              n2971 = Greater?(x=w3991, y=1) -> (0:w3987:bool)
            }
            n2972 = local write "String 29"(w3968) -> ()
            n2973 = Search and Replace String(input string=w3968, search string=".duf", replace string=".dgf" ("replace string (\"\")")) -> (result string=→"String Indicator 4":string)  [unwired: 5 in, 3 out]
            n2974 = Match Pattern(string=w3983, regular expression=".dwm") -> (before substring=w3967:string)  [unwired: 1 in, 3 out]
            "String Indicator" <- w3967
            n2975 = Match Pattern(string=w3968, regular expression=".dwm" ("substring (\"\")")) -> (before substring=w3969:string)  [unwired: 1 in, 3 out]
            "String Indicator 3" <- w3969
            n2976 = local write "TITTLE 2"(w3967) -> ()
            n2977 = String To Path(string=w3969) -> (path=w3976:path)
            "path" <- w3976
            n2978 = call <vilib>:"Read Characters From File.vi"("file path (dialog if empty)"=w3976, "start of read offset (chars.:0)"=60 ("start of read offset (chars.: 0)")) -> ("character string"=→"String Indicator 2":string)  [unwired: 4 in, 3 out]
          }
        }
        n2979 = call <vilib>:"Query Available Printers.vi"() -> ("system configured printers"=w3668:string[])  [unwired: 9 in, 2 out]
        "System Configured Printers 2" <- w3668
        n2980 = local read "OK Button 16"() -> (w3665:bool)
        n2981 = case shown="True" "OK Button 16" {
          frame False {
          }
          frame True {
            n2982 = stacked-sequence {
              frame #0 {
                n2983 = local read "Numeric 16"() -> (w3993:i32)
                n2984 = local write "Numeric 10"(w3993) -> ()
              }
              frame #1 {
                n2985 = local read "S.NO"() -> (→"s.NO":string)
                n2986 = local read "String 29"() -> (w3997:string)
                n2987 = String To Path(string=w3997) -> (path=w3996:path)
                n2988 = Open/Create/Replace File "Open File"(file path (use dialog)=w3996) -> (refnum out=w3998:refnum<file>)  [unwired: 5 in, 2 out]
                n2989 = for {
                  N: 16 -> [_]
                  tunnel: w3998 -> [w4005]
                  i -> [w4001]
                  (unwired) TRUE ("line mode (F)")
                  n2990 = Read from Text File "Read File"(file (use dialog)=w4005) -> (text=w3999:string)  [unwired: 3 in, 3 out]
                  n2991 = Match Pattern(string=w3999, regular expression="(") -> (after substring=w4004:string)  [unwired: 1 in, 3 out]
                  n2992 = Match Pattern(string=w4004, regular expression=")") -> (before substring=w4000:string)  [unwired: 1 in, 3 out]
                  n2993 = case shown="1" w4001 {
                    tunnel: w4000 -> [w4006 w4007 _ _ w4008 w4009 w4010 w4012 w4014 w4016 w4018 w4020 w4022 w4024 _]
                    tunnel: w3999 -> [_ _ _ _ _ _ _ _ _ _ _ _ _ _ _]
                    frame 0 {
                      "TITTLE" <- w4006
                    }
                    frame 1 {
                      "Sample ID" <- w4007
                    }
                    frame 2 {
                    }
                    frame 3 {
                    }
                    frame 4 {
                      "Test Date" <- w4008
                    }
                    frame 5 {
                      "Tested by" <- w4009
                    }
                    frame 6 {
                      n2994 = Fract/Exp String To Number(string=w4010) -> (number=→"Humidity before test 2":dbl)  [unwired: 3 in, 1 out]
                    }
                    frame 7 {
                      n2995 = Fract/Exp String To Number(string=w4012) -> (number=→"Temperature before test 2":dbl)  [unwired: 3 in, 1 out]
                    }
                    frame 8 {
                      n2996 = Fract/Exp String To Number(string=w4014) -> (number=→"Humidity after test 2":dbl)  [unwired: 3 in, 1 out]
                    }
                    frame 9 {
                      n2997 = Fract/Exp String To Number(string=w4016) -> (number=→"Temperature after test 2":dbl)  [unwired: 3 in, 1 out]
                    }
                    frame 10 {
                      n2998 = Fract/Exp String To Number(string=w4018) -> (number=→"MWSD 2":dbl)  [unwired: 3 in, 1 out]
                    }
                    frame 11 {
                      n2999 = Fract/Exp String To Number(string=w4020) -> (number=→"AVP 2":dbl)  [unwired: 3 in, 1 out]
                    }
                    frame 12 {
                      n3000 = Fract/Exp String To Number(string=w4022) -> (number=→"HCF 2":dbl)  [unwired: 3 in, 1 out]
                    }
                    frame 13 {
                      n3001 = Fract/Exp String To Number(string=w4024) -> (number=→"WS1.4 2":dbl)  [unwired: 3 in, 1 out]
                    }
                    frame 14, Default {
                    }
                  }
                }
              }
              frame #2 {
              }
            }
            n3002 = local write "OK Button 16"(FALSE ("OK Button 13")) -> ()
          }
        }
        n3003 = Index Array(array=w3668, index="Select Printer 3") -> (element=w3670:string)
        "Selected Printer" <- w3670
        n3004 = case shown="True" w3665 {
          frame False {
          }
          frame True {
            n3005 = flat-sequence {
              frame #0 {
              }
              frame #1 {
                n3006 = Wait (ms)(milliseconds to wait=u32 100) -> ()  [unwired: 1 out]
              }
              frame #2 {
                n3007 = local write "OK Button 16"(FALSE ("Print 3")) -> ()
              }
            }
          }
        }
        n3008 = case shown="True" "Print" {
          tunnel: w3670 -> [_ w3962]
          frame False {
          }
          frame True {
            (unwired) i16 6 ("width (-)")
            (unwired) "TESTED BY : "
            (unwired) "TESTED DATE :"
            (unwired) "SAMPLE ID : "
            (unwired) "SAMPLE DESIGN : "
            w3920 = "\r"
            w3937 = "\r"
            # "add image"
            n3009 = local read "Sample ID"() -> (w3910:string)
            n3010 = local read "Tested by"() -> (w3913:string)
            n3011 = local read "String 34"() -> (w3900:string)
            n3012 = local read "String 45"() -> (w3880:string)
            n3013 = local read "String 35"() -> (w3895:string)
            n3014 = local read "String 37"() -> (w3893:string)
            n3015 = local read "String 32"() -> (w3915:string)
            n3016 = local read "String 36"() -> (w3890:string)
            n3017 = local read "String 31"() -> (w3914:string)
            n3018 = local read "Test Date"() -> (w3911:string)
            n3019 = local read "String 33"() -> (w3916:string)
            n3020 = local read "String 38"() -> (w3886:string)
            n3021 = local read "String 39"() -> (w3883:string)
            n3022 = local write "Print"(FALSE ("Print FF")) -> ()
            n3023 = local read "S 39"() -> (w3898:string)
            n3024 = local read "S 38"() -> (w3905:string)
            n3025 = local read "Temperature before test 2"() -> (w3936:dbl)
            n3026 = local read "Temperature after test 2"() -> (w3926:dbl)
            n3027 = local read "Humidity before test 2"() -> (w3951:dbl)
            n3028 = local read "Humidity after test 2"() -> (w3935:dbl)
            n3029 = local read "MWSD 2"() -> (w3940:dbl)
            n3030 = local read "WS1.4 2"() -> (w3918:dbl)
            n3031 = Concatenate Strings("2)" ("string"), w3900) -> (w3901:string)
            n3032 = Concatenate Strings("3)" ("string"), w3898) -> (w3899:string)
            n3033 = Concatenate Strings("1)" ("string"), w3905) -> (w3904:string)
            n3034 = Concatenate Strings("4)" ("string"), w3895) -> (w3896:string)
            n3035 = Concatenate Strings("5)" ("string"), w3893) -> (w3892:string)
            n3036 = Concatenate Strings("6)" ("string"), w3890) -> (w3889:string)
            n3037 = Concatenate Strings("7)" ("string"), w3886) -> (w3887:string)
            n3038 = Concatenate Strings("8)" ("string"), w3883) -> (w3884:string)
            n3039 = local read "HCF 2"() -> (w3922:dbl)
            n3040 = local read "AVP 2"() -> (w3939:dbl)
            n3041 = local read "s.NO"() -> (w3881:string)
            n3042 = call <vilib>:"New Report.vi"("report type"=enum16{"Standard Report", "HTML"}."Standard Report") -> ("report out"=w3960:refnum<class "NI_report.lvclass">, "error out"=w3959:errorcluster)  [unwired: 13 in]
            n3043 = local read "TITTLE"() -> (w3912:string)
            n3044 = Concatenate Strings(w3937, w3880, w3881, w3937, w3915, w3910, w3937, w3914, w3911, w3937, w3916, w3913, w3937) -> (w3930:string)
            "test by" <- w3930
            n3045 = Number To Fractional String(number=w3936, width (-)=i16 6, precision (6)=i16 2) -> (F-format string=w3925:string)  [unwired: 1 in]
            n3046 = Number To Fractional String(number=w3935, width (-)=i16 6, precision (6)=i16 2) -> (F-format string=w3938:string)  [unwired: 1 in]
            n3047 = Number To Fractional String(number=w3951, width (-)=i16 6, precision (6)=i16 2) -> (F-format string=w3956:string)  [unwired: 1 in]
            n3048 = Number To Fractional String(number=w3940, width (-)=i16 6, precision (6)=i16 2) -> (F-format string=w3942:string)  [unwired: 1 in]
            n3049 = Number To Fractional String(number=w3926, width (-)=i16 6, precision (6)=i16 2) -> (F-format string=w3927:string)  [unwired: 1 in]
            n3050 = Number To Fractional String(number=w3939, width (-)=i16 6, precision (6)=i16 2) -> (F-format string=w3941:string)  [unwired: 1 in]
            n3051 = Number To Fractional String(number=w3922, width (-)=i16 6, precision (6)=i16 2) -> (F-format string=w3921:string)  [unwired: 1 in]
            n3052 = Number To Fractional String(number=w3918, precision (6)=i16 2) -> (F-format string=w3917:string)  [unwired: 2 in]
            n3053 = call-dynamic "Set Report Header Text.vi"("report in"=w3960, "center header text"=w3912, "error in (no error)"=w3959) -> ("report out"=w3931:refnum<class "NI_report.lvclass">, "error out"=w3932:errorcluster)  [unwired: 11 in]
            n3054 = Concatenate Strings(w3920, w3904, w3956, w3920, w3901, w3925, w3920, w3899, w3938, w3920, w3896, w3927, w3920, w3892, w3942, w3920, w3889, w3941, w3920, w3887, w3921, w3920, w3884, w3917) -> (w3908:string)
            "export 2" <- w3908
            n3055 = call-poly <vilib>:"Append Report Text.vi"("report in"=w3931, "text"=w3930, "error in (no error)"=w3932) -> ("report out"=w3934:refnum<class "NI_report.lvclass">, "error out"=w3933:errorcluster)  [unwired: 9 in, 2 out]
            n3056 = local read "test by"() -> (w3907:string)
            n3057 = local read "TITTLE"() -> (w3909:string)
            n3058 = call-poly <vilib>:"Append Report Text.vi"("report in"=w3934, "error in (no error)"=w3933) -> ("report out"=w3955:refnum<class "NI_report.lvclass">, "error out"=w3953:errorcluster)  [unwired: 10 in, 2 out]
            n3059 = Concatenate Strings(w3909, w3908, w3907) -> (→"output":string)
            n3060 = call-poly <vilib>:"Append Report Text.vi"("report in"=w3955, "text"=w3908, "error in (no error)"=w3953) -> ("report out"=w3954:refnum<class "NI_report.lvclass">, "error out"=w3952:errorcluster)  [unwired: 9 in, 2 out]
            n3061 = call-dynamic "Print Report.vi"("report in"=w3954, "printer name (default)"=w3962, "error in (no error)"=w3952) -> ("report out"=w3964:refnum<class "NI_report.lvclass">, "error out"=w3965:errorcluster)  [unwired: 11 in]
            n3062 = call-dynamic "Dispose Report.vi"("report in"=w3964, "error in (no error)"=w3965) -> ()  [unwired: 13 in, 1 out]
          }
        }
        n3063 = case shown="True" "Print 2" {
          frame False {
          }
          frame True {
            n3064 = flat-sequence {
              frame #0 {
                n3065 = local read "s.NO"() -> (→"s.NO 2":string)
                n3066 = Wait (ms)(milliseconds to wait=u32 20) -> ()  [unwired: 1 out]
                n3067 = local read "Sample ID  3"() -> (→"Sample ID  6":string)
                n3068 = local read "Sample ID  4"() -> (→"Sample ID  7":string)
                n3069 = local read "Sample ID"() -> (→"Sample ID  2":string)
                n3070 = local read "Tested by"() -> (→"Tested by 2":string)
                n3071 = local read "Test Date"() -> (→"Test Date 2":string)
                n3072 = local read "Humidity after test 3"() -> (→"Humidity after test 4":dbl)
                n3073 = local read "Ref A Test Date :"() -> (→"TITTLE 4":string)
                n3074 = local read "Temperature before test 3"() -> (w3787:dbl)
